vi "Write CAN FIFO.vi"(6 "FIFO Timestamps":T1, 8 "error in (no error)":errorcluster, 9 "Timeout (ms)":i32, 10 "Data":u8[](array[numeric]) format="%.0x", 11 "CIFTag in":refnum<class "CIF_NIChn_FifoCAN.lvclass">) -> (0 "error out":errorcluster, 1 "timed out?":bool, 3 "CIFTag out":refnum<class "CIF_NIChn_FifoCAN.lvclass">)   [LabVIEW 2021, in "CIF_NIChn_FifoCAN.lvclass"]
uses:
  CIF_NIChn_FifoCAN.lvclass
  ChannelCommon/typedef/TimeStamps.ctl
  CIF_NIChn_FifoCAN.lvclass/CIF_NIChn_FifoCAN.ctl
  ChannelCommon/ChannelCommon.lvlib
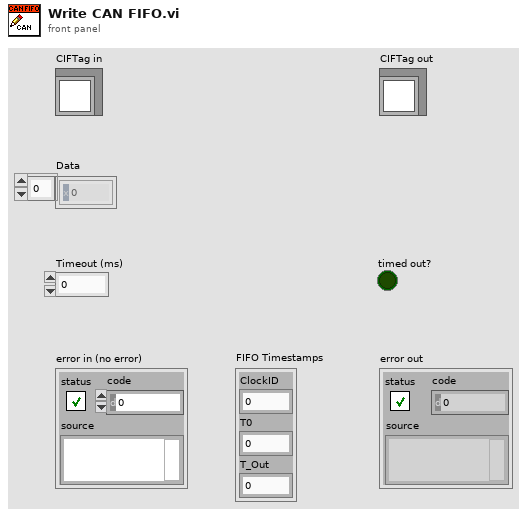
[diagram p1: front panel]
types:
  T1 = typedef "ChannelCommon.lvlib/TimeStamps.ctl" = cluster{"ClockID":u8, "T0":i64, "T_Out":i64}
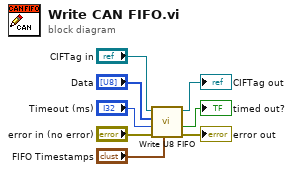
[diagram p0: block diagram]
diagram:
  n1 = call-dynamic "Write U8 FIFO.vi"("FIFO Timestamps"="FIFO Timestamps", "error in (no error)"="error in (no error)", "Timeout (ms)"="Timeout (ms)", "Data in"="Data", "CIFFIFO in"="CIFTag in") -> ("error out"=→"error out":errorcluster, "timed out?"=→"timed out?":bool, "CIFFIFO out"=→"CIFTag out":refnum<class "CIF_NIChn_FifoCAN.lvclass">)  [unwired: 3 in, 1 out]
